vi "usb set Power Enable LV.vi"(8 "error in (no error)":errorcluster, 9 "port":i32, 10 "result":cluster{"value":i32, "error":i32}, 11 "id":i32) -> (0 "error out":errorcluster, 2 "result out":cluster{"value":i32, "error":i32}, 3 "id out":i32)   [LabVIEW 2015, in "BrainStem4LabView.lvlib"]
doc: "__declspec(dllexport) void __stdcall usb_setPowerEnable_LV(int* id, struct Result* result, int port);"
uses:
  BrainStem4LabView.lvlib
  LabViewTesting.dll
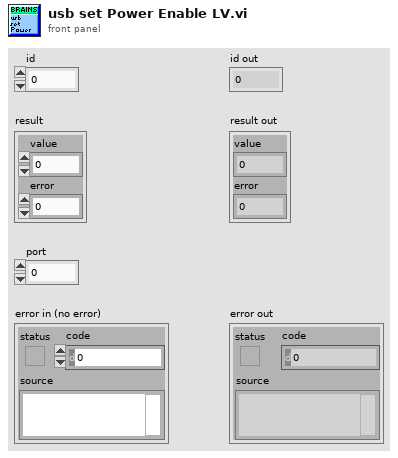
[diagram p1: front panel]
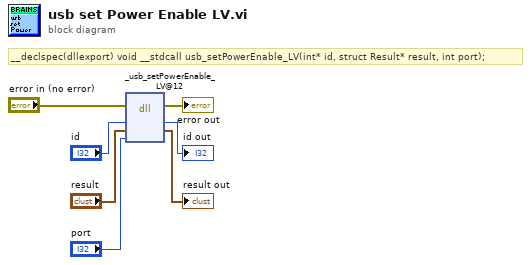
[diagram p0: block diagram]
diagram:
  # "__declspec(dllexport) void __stdcall usb_setPowerEnable_LV(int* id, struct Result* result, int port);"
  n1 = dll-call lib="C:/Users/Acroname_User/development/acroname/software/acroname/aSource/LabVIEW/LabView_BS_Project/BrainStem_DLL_Import/LabViewTesting.*" fn="_usb_setPowerEnable_LV@12"(error in="error in (no error)", "id"="id", "result"="result", "port"="port") -> (error out=→"error out":errorcluster, "id"=→"id out":i32, "result"=→"result out":cluster{"value":i32, "error":i32})  [unwired: 4 in, 1 out]
